vi "selection.vi"(8 "Error In":errorcluster, 11 "GenAlg_data":T1) -> (0 "Error Out":errorcluster, 3 "GenAlg_data-out":T1)   [LabVIEW 2016]
uses:
  TypeDefs/GenAlg_data.ctl
  TypeDefs/basic_config.ctl
  TypeDefs/element.ctl
  TypeDefs/geration_data.ctl
  TypeDefs/selection_data.ctl
  TypeDefs/SimulatedAnnealing_data.ctl
  TypeDefs/multi_eval_data.ctl
  TypeDefs/termination_data.ctl
  <userlib>/_OpenG.lib/array/array.llb/Sort 1D Array (DBL)__ogtk.vi
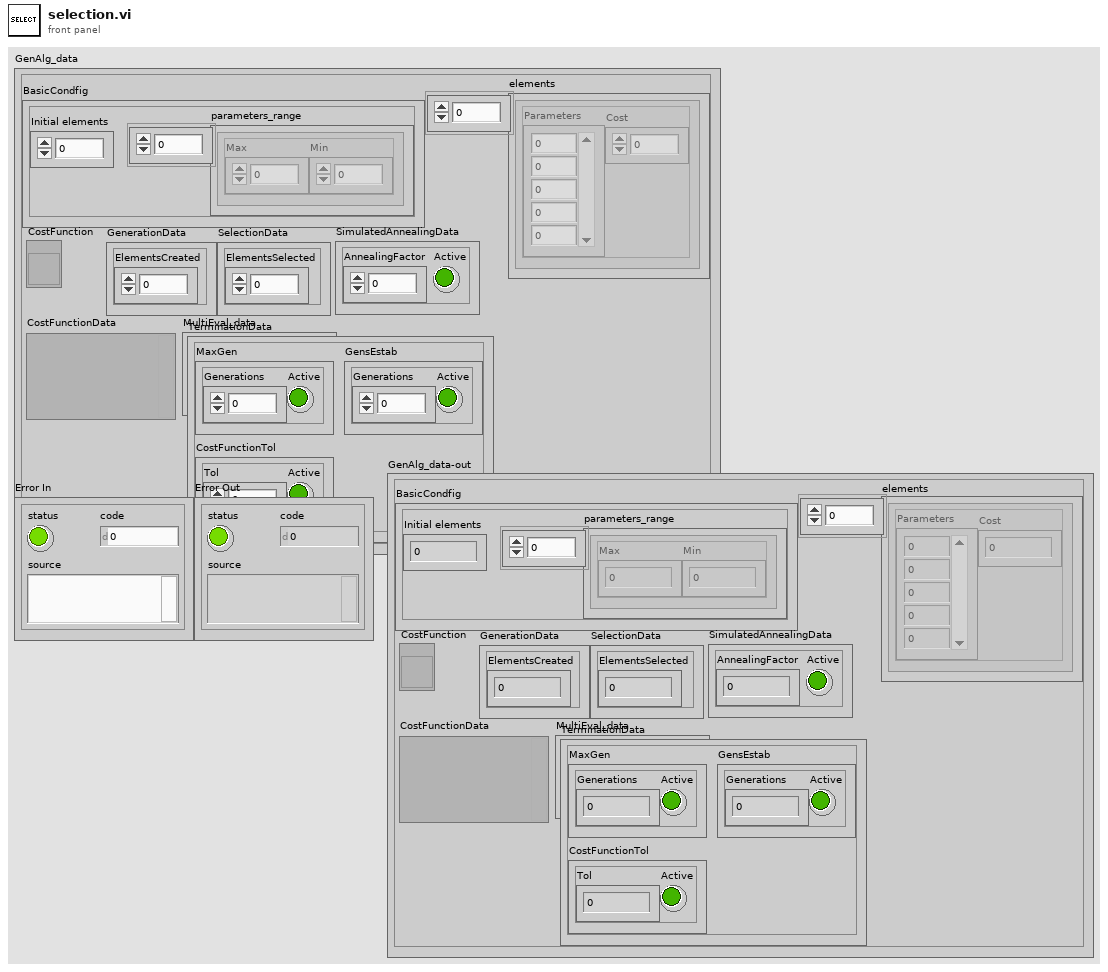
[diagram p1: front panel]
types:
  T1 = typedef "GenAlg_data.ctl" = cluster{"BasicCondfig":T2, "elements":T3[], "CostFunction":refnum<vi>, "GenerationData":T4, "SelectionData":T5, "SimulatedAnnealingData":T6, "CostFunctionData":variant, "MultiEval_data":T7, "TerminationData":T8}
  T2 = typedef "basic_config.ctl" = cluster{"parameters_range":cluster{"Max":dbl, "Min":dbl}[], "Initial elements":i32}
  T3 = typedef "element.ctl" = cluster{"Parameters":dbl[], "Cost":dbl}
  T4 = typedef "geration_data.ctl" = cluster{"ElementsCreated":i32}
  T5 = typedef "selection_data.ctl" = cluster{"ElementsSelected":i32}
  T6 = typedef "SimulatedAnnealing_data.ctl" = cluster{"AnnealingFactor":dbl, "Active":bool}
  T7 = typedef "multi_eval_data.ctl" = cluster{"Active":bool, "MultiEvalFunction":refnum<vi>}
  T8 = typedef "termination_data.ctl" = cluster{"MaxGen":cluster{"Generations":i32, "Active":bool}, "CostFunctionTol":cluster{"Tol":dbl, "Active":bool}, "GensEstab":cluster{"Generations":i32, "Active":bool}}
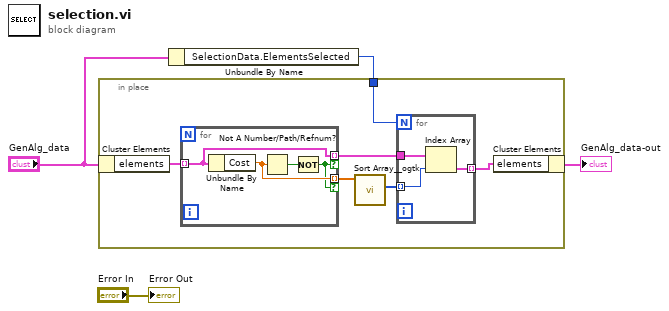
[diagram p0: block diagram]
diagram:
  n1 = Unbundle By Name("GenAlg_data") -> ("SelectionData.ElementsSelected"=w1:i32)
  n2 = in-place {
    in-place-border: w1 -> [w6]
    n3 = in-place-cluster #1("GenAlg_data") -> ("elements"=w10:T3[])
    n4 = for {
      tunnel: w10 -> [w15] mode=indexing
      tunnel: [w17] -> w5 mode=indexing if=w14
      tunnel: [w15] -> w9 mode=indexing if=w14
      n5 = Unbundle By Name(w15) -> ("Cost"=w17:dbl)
      n6 = Not A Number/Path/Refnum?(number/path/refnum=w17) -> (NaN/Path/Refnum?=w16:bool)
      n7 = Not(x=w16) -> (.not. x?=w14:bool)
    }
    n8 = call-poly <userlib>:"Sort Array__ogtk.vi"("Array in"=w5) -> ("Sorted Pointers"=w8:i32[])  [unwired: 9 in, 1 out]
    n9 = for {
      N: w6 -> [_]
      tunnel: w9 -> [w13]
      tunnel: w8 -> [w12] mode=indexing
      tunnel: [w11] -> w7 mode=indexing
      n10 = Index Array(array=w13, index=w12) -> (element=w11:T3)
    }
    n11 = in-place-cluster #1("elements"=w7) -> (→"GenAlg_data-out":T1)
  }
  "Error Out" <- "Error In"
